vi "Dashboard Main.vi"() -> ()   [LabVIEW 2014]
uses:
  <vilib>/event_ctls.llb/eventvkey.ctl
  <vilib>/Rock Robotics/WPI/Dashboard/WPI_DashboardLogging Global.vi
  <vilib>/Rock Robotics/Network Tables/SD Write Number.vi
  <vilib>/Rock Robotics/Network Tables/SD Read Number.vi
  <vilib>/Utility/config.llb/Write Key (String).vi
  <vilib>/Utility/config.llb/Write Key (I32).vi
  <vilib>/Utility/config.llb/NI_LVConfig.lvlib
panel:
  out "Numeric Array":dbl[](array[numeric])
  in  "TCP":refnum<k5>
  in  "Rec Mode":enum32{"Stop", "Record", "Playback"}(radio)
  in  "Vision":u16(ring) items=["Camera Off", "USB Camera SW", "USB Camera HW", "IP Camera"]
  out "Camera IP":string
  out "Image Message":string="Timeout in Camera Communications"
  in  "Dashboard Tab":T1(tab)
  out "pot":dbl(slide) scale=0.0..30.0
  in  "LED_Off":u32(colorbox)=65282
  in  "Camera Settings":T2={"Frame Rate"=30, "Compression"=30, "Size"=1} {"Frame Rate" scale=1.0..30.0; "Size" items=["640x480", "320x240", "160x120"]}
  out "MotorChart R":cluster{"Numeric":dbl, "Numeric":dbl}(graph)
  out "MotorChart L":T3(graph)
  out "MotorSliders R":cluster{"MotorSlide1":dbl, "MotorSlide2":dbl} {"MotorSlide2" scale=-1.0..1.0 scale format="%#_2e"; "MotorSlide1" scale=-1.0..1.0 scale format="%#_2e"}
  out "MotorSliders L":T4 {"MotorSlide4 2" scale=0.0..14.0 scale format="%#_2e"; "MotorSlide2" scale=-1.0..1.0 scale format="%#_2e"; "MotorSlide1" scale=-1.0..1.0 scale format="%#_2e"}
  out "Gyro":dbl(knob) scale=0.0..360.0
  out "JS1 Z":dbl(slide) scale=-1.0..1.0 scale format="%#_2e"
  out "JS1 Graph":cluster{"X":dbl, "Y":dbl}[](graph)
  out "JS1 Buttons":T5
  out "JS2 Z":dbl(slide) scale=-1.0..1.0 scale format="%#_2e"
  out "JS2 Graph":cluster{"X":dbl, "Y":dbl}[](graph)
  out "JS2 Buttons":T5
  out "Mode":T6(ring)=enum."Auto Disabled"
  in  "DB Camera Config":bool
  out "fps":dbl format="%#.1g"
  out "Mbps":dbl format="%#.1g"
  out "Mbps 2":bool
  in  "LED_On":u32(colorbox)=1535
  in  "DB/String 9":string
  in  "DB/String 8":string
  in  "DB/String 7":string
  in  "DB/String 6":string
  in  "DB/String 5":string
  in  "DB/String 4":string
  in  "DB/String 3":string
  in  "DB/String 2":string
  in  "DB/String 1":string
  in  "DB/String 0":string
  in  "DB/Slider 0":dbl(slide) scale=0.0..5.0
  in  "DB/Slider 1":dbl(slide) scale=0.0..5.0
  in  "DB/Slider 2":dbl(slide) scale=0.0..5.0
  in  "DB/Slider 3":dbl(slide) scale=0.0..5.0
  out "DB/LED 3":bool
  out "DB/LED 2":bool
  out "DB/LED 1":bool
  out "DB/LED 0":bool
  in  "DB/Button 3":bool
  in  "DB/Button 2":bool
  in  "DB/Button 1":bool
  in  "DB/Button 0":bool caption="New Name"
  in  "Test Slider":dbl(slide) scale=0.0..100.0 scale format="%#_3g"
  in  "On/Off":bool caption="Solenoid"
  in  "Test Name":u16(ring) items=["Select the test to run...", "Example Test", "-------------------------------", "List of tests is built in robot code.", "Replace with your own automated tests."]
  in  "Test Tree":string(tree)
  in  "Motor":cluster{"Value":dbl, "Enable":bool} {"Value" scale=-1.0..1.0 scale format="%#_3g"}
  out "Progress":T7 {"Test Progress" scale=0.0..100.0}
  in  "Rev/Fwd":cluster{"Forward":bool, "Reverse":bool}
  in  "Test Ring":u16(ring) items=["Monochrome", "Color"]
  in  "Listbox":i32(listbox)
  out "Tree":string(tree)
  out "Camera Image":T8(plugin-control)
  out "Boolean":bool
  # "Left"
  # "Front"
  # "Right"
  # "Battery"
  # "This tab is a great place for autonomous settings and robot-specific values.\nPlace controls and indicators inside this tab and match name to\nDashboard Variables on robot. You can also delete this comment."
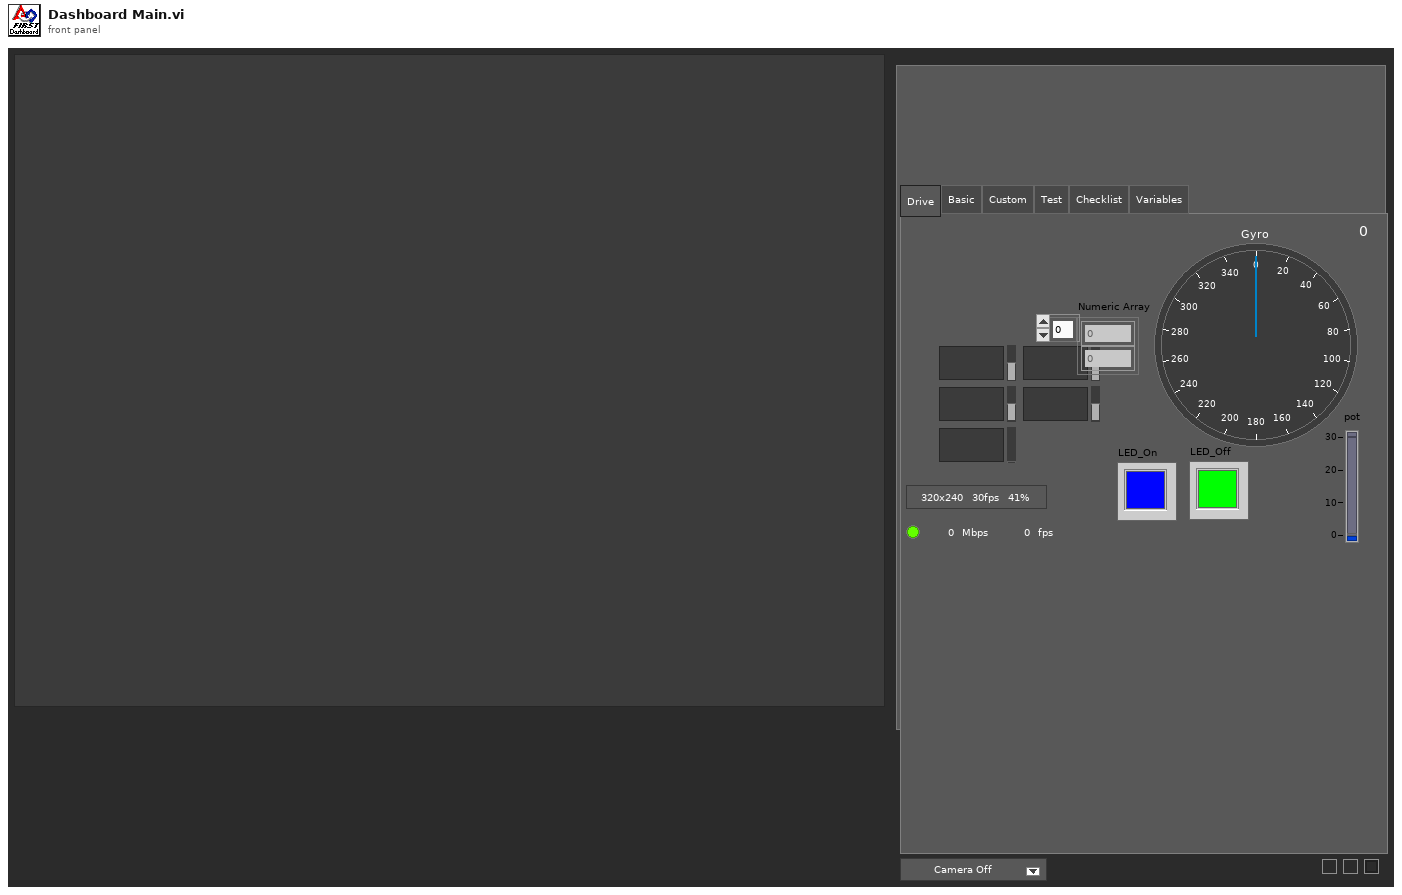
[diagram p1: front panel]
types:
  T1 = enum32{"Drive", "Basic", "Custom", "Test", "Checklist", "Variables"}
  T2 = cluster{"Frame Rate":i32, "Compression":i32, "Size":u16}
  T3 = cluster{"Numeric":dbl, "Numeric":dbl, "Battery V":dbl}
  T4 = cluster{"MotorSlide1":dbl, "MotorSlide2":dbl, "MotorSlide4 2":dbl}
  T5 = cluster{bool, bool, bool, bool, bool, bool, bool, bool, bool, bool, bool, bool}
  T6 = enum8{"Tele-Op Disabled", "Tele-Op Enabled", "Auto Disabled", "Auto Enabled", "Test Disabled", "Test Enabled", "Disconnected", "No Code", "E-Stop"}
  T7 = cluster{"Test Progress":u8, "Test Progress Text":string}
  T8 = typedef "IMAQ Image.ctl" = refnum<image>
  T9 = typedef "Image Type" = u32
  T10 = cluster{"Camera Image":refnum<vi>, "Dashboard Tab":refnum<vi>, "Boolean":refnum<vi>, "Vision":refnum<vi>, "Rec Mode":refnum<vi>, "Test Slider":refnum<vi>, "On/Off ":refnum<vi>, "Test Ring":refnum<vi>, "Rev/Fwd":refnum<vi>, "Test Name":refnum<vi>, "Motor":refnum<vi>, "Progress":refnum<vi>, "CheckList":refnum<vi>, "Tree":refnum<vi>, "Test Tree":refnum<vi>}
  T11 = cluster{"Error Strings":string, "Disable Counts":cluster{u16, u16}, "Rail Faults":cluster{u16, u16, u16}, "Robot IP":string, "DB Mode":u8, "Event Info":cluster{"Name":string, "Type":u8, "Number":u16, "Replay":u8}, "Camera Addr":string}
  T12 = cluster{"Storage":cluster{"Disk Free":u64, "RAM Block":u32, "RAM free":u32}, "CPU Utilization":cluster{"CPU % ISR":sgl, "CPU % Time Crit":sgl, "CPU % Timed Str":sgl, "CPU % High":sgl, "CPU % Above":sgl, "CPU % Normal":sgl, "CPU % Low":sgl}, "CAN":cluster{"% Bus Utilization":sgl, "Bus Off Cnt":u32, "TX_FIFO Full Cnt":u32, "Receive Error Cnt":u8, "Transmit Error Cnt":u8}, "HID":cluster{"HID Outputs":u32, "Rumble Low":u16, "Rumble High":u16}[]}
  T13 = cluster{"Status bits":cluster{"Test Mode":bool, "Autonomous":bool, "Enabled":bool, "Code Start":bool, "Brownout":bool, "Reserved 2":bool, "Reserved 3":bool, "E-Stop":bool}, "Code Trace":cluster{"Disabled":bool, "TeleOp":bool, "Auto":bool, "Test":bool}, "Controller Type":enum16{"unknown", "cRIO", "roboRio"}, "Code?":enum16{"unknown", "noCode", "code"}, "Battery V":dbl}
  T14 = cluster{"Control Bits":cluster{"TestMode":bool, "Autonomous":bool, "Enabled":bool, "FMS Present":bool, bool, bool, bool, "E-Stop":bool}, "Team Station ":u8, "Countdown":sgl, "Joystick Values":cluster{"Axes":dbl[], "Buttons":bool[], "POVs":i16[]}[]}
  T15 = cluster{"Axes":dbl[], "Buttons":bool[], "POVs":i16[]}[]
  T16 = cluster{"Axes":dbl[], "Buttons":bool[], "POVs":i16[]}
  T17 = cluster{"Buttons[0]":bool, "Buttons[1]":bool, "Buttons[2]":bool, "Buttons[3]":bool, "Buttons[4]":bool, "Buttons[5]":bool, "Buttons[6]":bool, "Buttons[7]":bool, "Buttons[8]":bool, "Buttons[9]":bool, "Buttons[10]":bool, "Buttons[11]":bool}
  T18 = typedef "NI_LVConfig.lvlib/Config Data RefNum.ctl" = refnum<k1>
  T19 = cluster{"Operation":enum16{"Update", "Clear"}, "Color Box":u32}[]
  T20 = typedef "eventvkey.ctl" = enum16{"ASCII", "Enter", "Return", "Shift", "Ctrl", "Alt", "Cmd", "Opt", "Caps", "NumLock", "Clear", "Break", "Up", "Down", "Left", "Right", "Insert", "Delete", "Home", "End", "PageUp", "PageDown", "Escape", "Help", "Pause", "ScrollLock", "F1", "F2", "F3", "F4", "F5", "F6", "F7", "F8", "F9", "F10", "F11", "F12", "F13", "F14", "F15", "F16", "F17", "F18", "F19", "F20", "F21", "F22", "F23", "F24", "Play", "VolumeUp", "VolumeDown", "Mute", "Two Byte Char"}
  T21 = cluster{"Image Size":bool, "Image Type":bool, "Pixel Value":bool, "ROI Information":bool, "Zoom Factor":bool}
  T22 = enum8{"Enabled", "Disabled", "Disabled and Grayed Out"}
  T23 = cluster{"Operation":enum16{"Update", "Clear"}, "Color Box":u32}
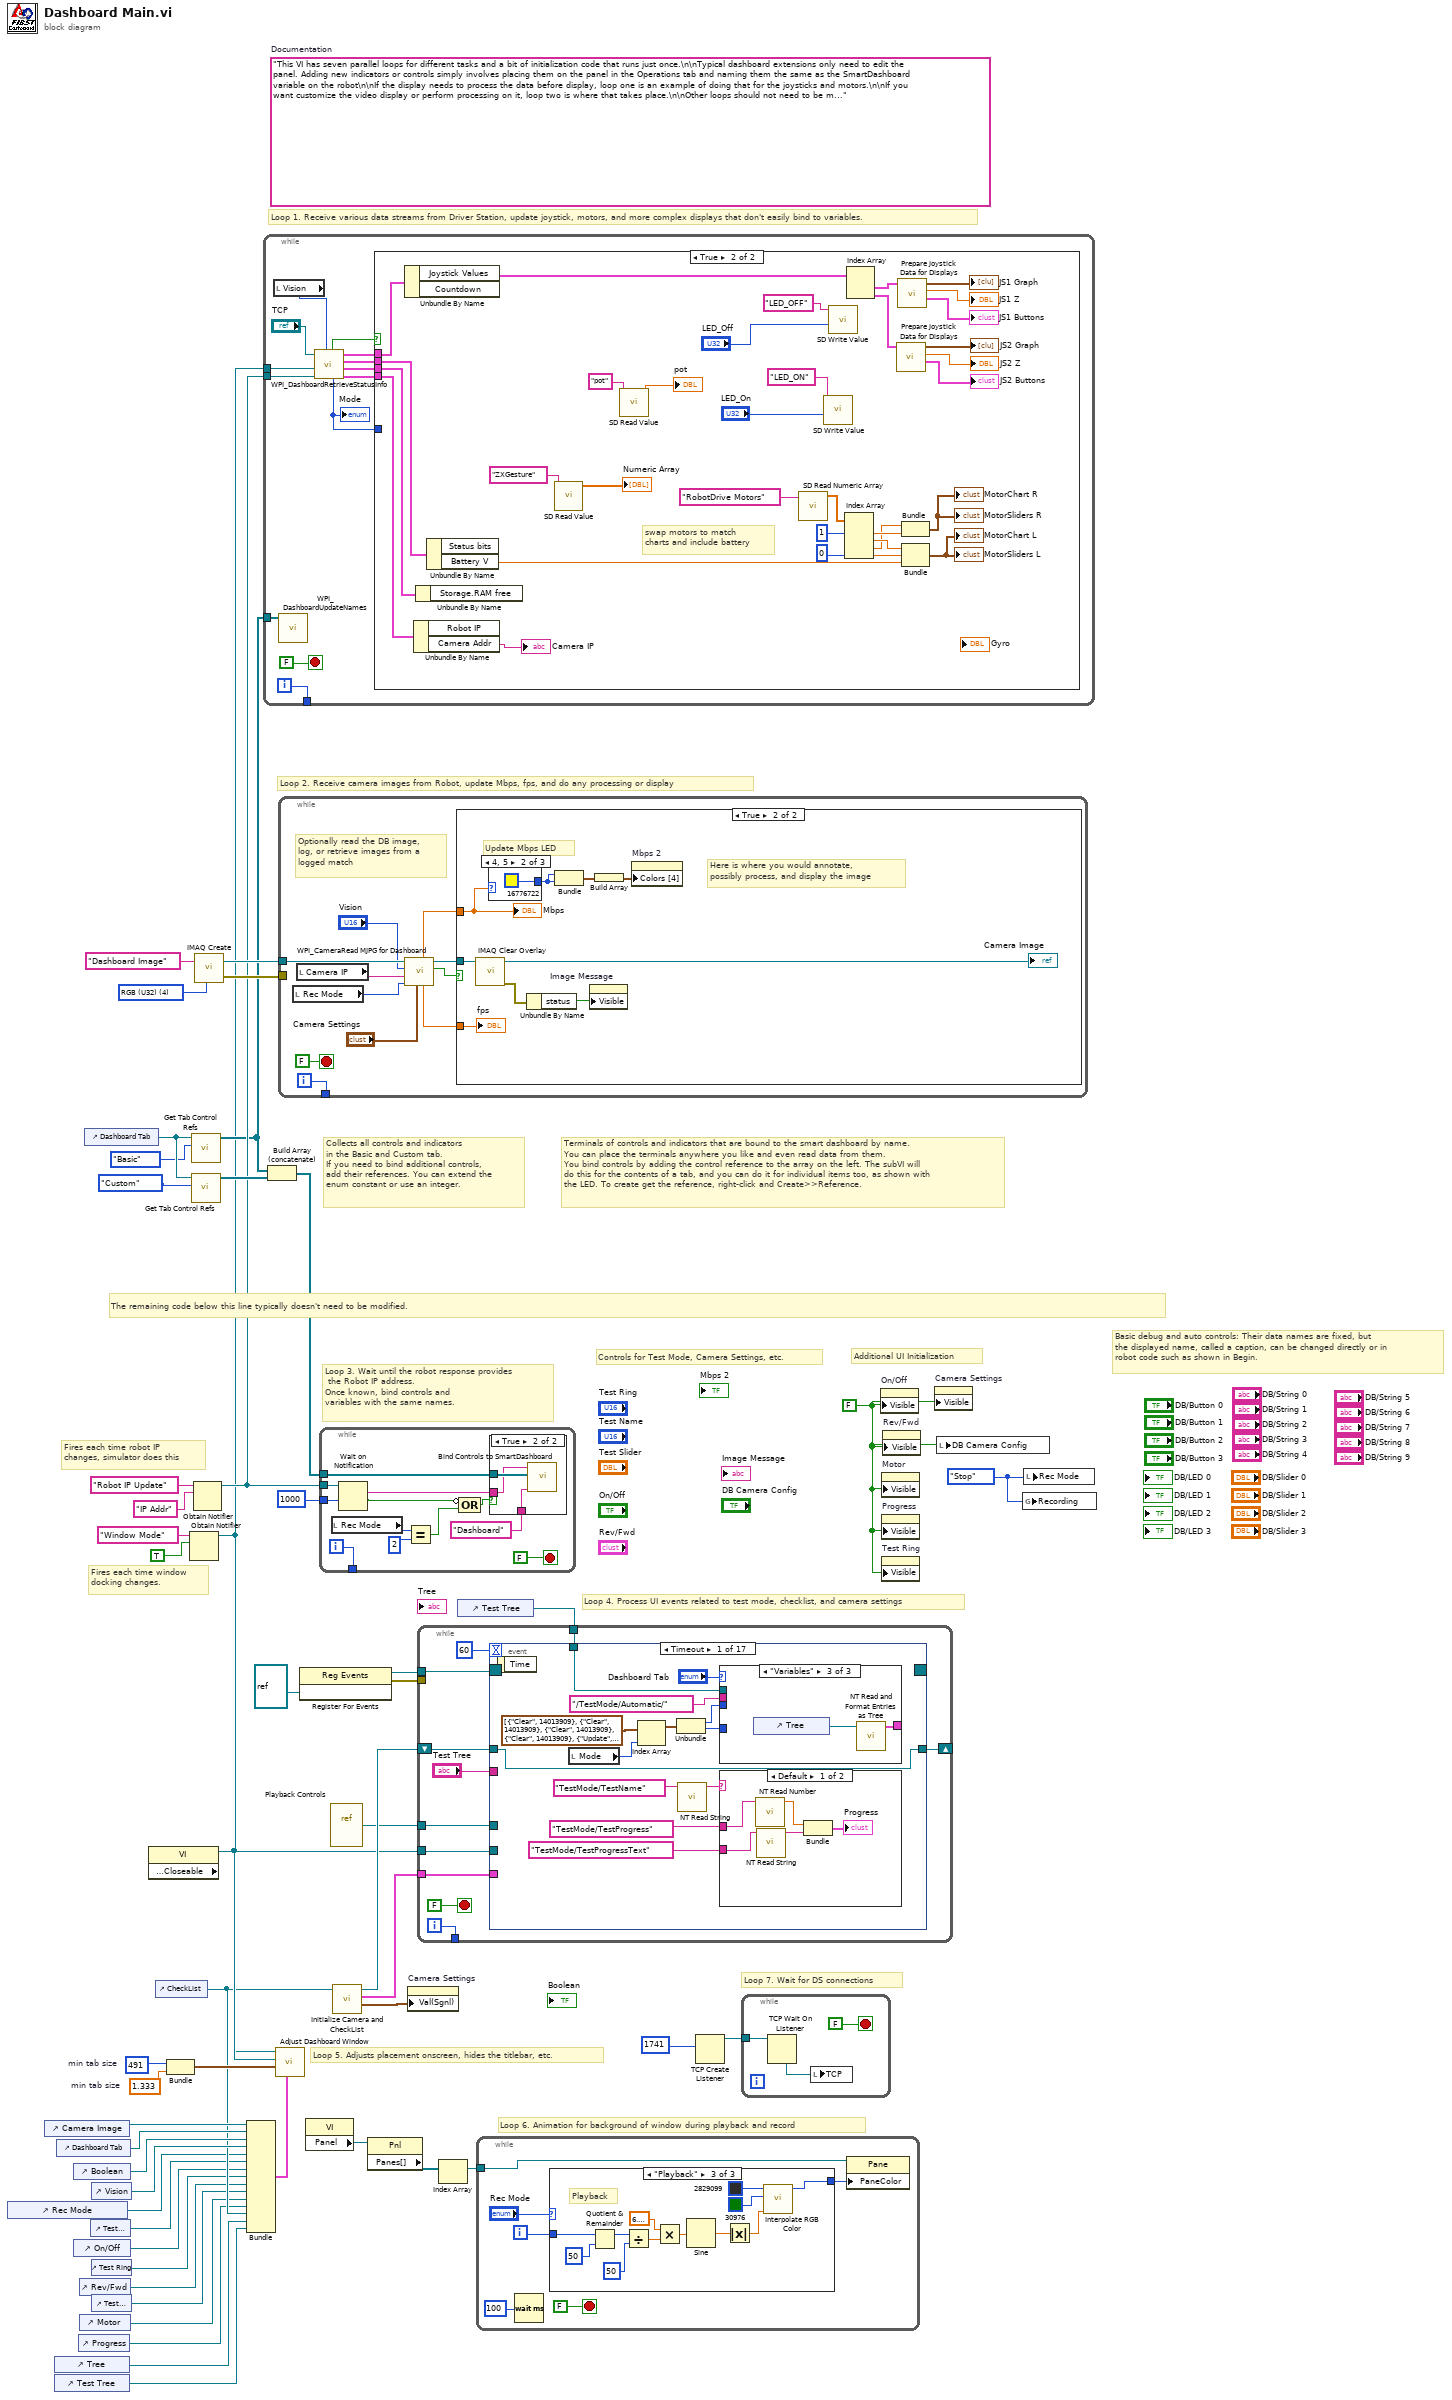
[diagram p0: block diagram]
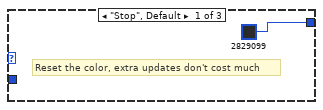
[diagram p3: hidden frame]
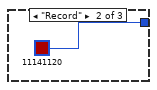
[diagram p4: hidden frame]
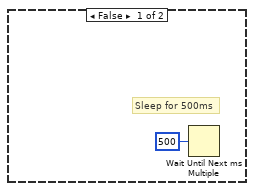
[diagram p6: hidden frame]
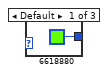
[diagram p7: hidden frame]
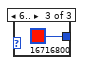
[diagram p8: hidden frame]
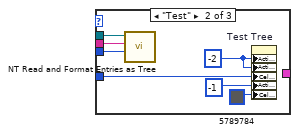
[diagram p10: hidden frame]
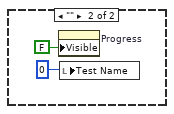
[diagram p11: hidden frame]
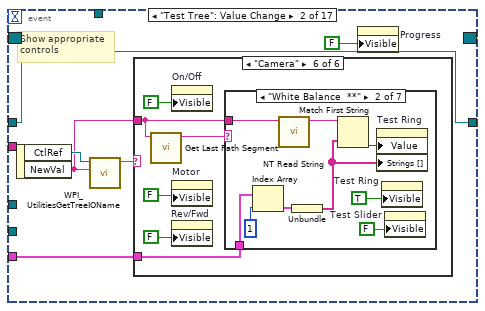
[diagram p12: hidden frame]
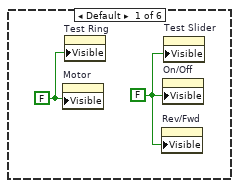
[diagram p13: hidden frame]
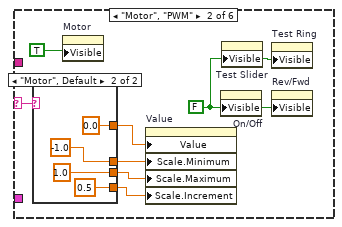
[diagram p14: hidden frame]
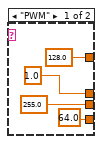
[diagram p15: hidden frame]
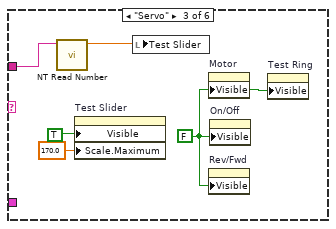
[diagram p16: hidden frame]
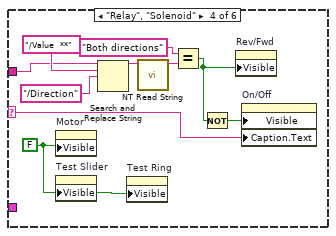
[diagram p17: hidden frame]
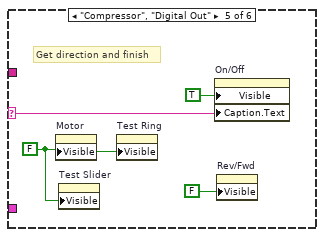
[diagram p18: hidden frame]
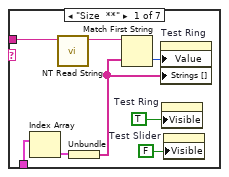
[diagram p19: hidden frame]
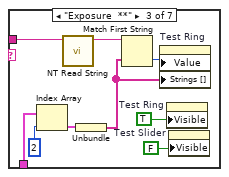
[diagram p20: hidden frame]
diagram:
  w24 = 491  # min tab size
  w23 = 1.333  # min tab size
  w32 = enum32{"Stop", "Record", "Playback"}."Stop" ("Rec Mode")
  w6 = FALSE ("Visible")
  (unwired) "This VI has seven parallel loops for different tasks and a bit of initialization code that runs just once.\n\nTypical dashboard extensions only need to edit the panel. Adding new indicators or controls simply involves placing them on the panel in the Operations tab and naming them the same as the SmartDashboard variable on the robot\n\nIf the display needs to process the data before display, loop one is an example of doing that for the joysticks and motors.\n\nIf you want customize the video display or perform processing on it, loop two is where that takes place.\n\nOther loops should not need to be modified. They are pretty standard, and document the task they perform."  # Documentation
  w52 = T9 4 items=["Grayscale (U8)", "Grayscale (I16)", "Grayscale (SGL)", "Complex (CSG)", "RGB (U32)", "HSL (U32)", "RGB (U64)"] ("Image Type")
  # "Loop 7. Wait for DS connections"
  # "Basic debug and auto controls: Their data names are fixed, but\nthe displayed name, called a caption, can be changed directly or in\nrobot code such as shown in Begin."
  # "Controls for Test Mode, Camera Settings, etc."
  # "Additional UI Initialization"
  # "Loop 6. Animation for background of window during playback and record"
  # "Fires each time robot IP\nchanges, simulator does this"
  # "Fires each time window\ndocking changes."
  # "Collects all controls and indicators\nin the Basic and Custom tab.\nIf you need to bind additional controls,\nadd their references. You can extend the\nenum constant or use an integer."
  # "The remaining code below this line typically doesn't need to be modified."
  # "Loop 4. Process UI events related to test mode, checklist, and camera settings"
  # "Terminals of controls and indicators that are bound to the smart dashboard by name.\nYou can place the terminals anywhere you like and even read data from them.\nYou bind controls by adding the control reference to the array on the left. The subVI will\ndo this for the contents of a tab, and you can do it for individual items too, as shown with\nthe LED. To create get the reference, right-click and Create>>Reference."
  # "Loop 3. Wait until the robot response provides\n the Robot IP address.\nOnce known, bind controls and\nvariables with the same names."
  # "Loop 5. Adjusts placement onscreen, hides the titlebar, etc."
  # "Loop 1. Receive various data streams from Driver Station, update joystick, motors, and more complex displays that don't easily bind to variables."
  # "Loop 2. Receive camera images from Robot, update Mbps, fps, and do any processing or display"
  n1 = control-ref of="Rec Mode"() -> (w12:refnum<vi>)
  n2 = control-ref of="Camera Image"() -> (w27:refnum<vi>)
  n3 = control-ref of="Tree"() -> (w16:refnum<vi>)
  n4 = control-ref of="Test Tree"() -> (w15:refnum<vi>)
  n5 = control-ref of="Dashboard Tab"() -> (w26:refnum<vi>)
  n6 = control-ref of="Boolean"() -> (w21:refnum<vi>)
  n7 = control-ref of="On/Off"() -> (w10:refnum<vi>)
  n8 = control-ref of="Progress"() -> (w7:refnum<vi>)
  n9 = control-ref of="Rev/Fwd"() -> (w8:refnum<vi>)
  n10 = control-ref of="Motor"() -> (w13:refnum<vi>)
  n11 = control-ref of="Dashboard Tab"() -> (w30:refnum<vi>)
  n12 = control-ref of="Test Slider"() -> (w11:refnum<vi>)
  n13 = control-ref of="Vision"() -> (w25:refnum<vi>)
  n14 = control-ref of="Test Ring"() -> (w9:refnum<vi>)
  n15 = control-ref of="Test Name"() -> (w14:refnum<vi>)
  n16 = property class="VI" props=["Front Panel.Closeable"]() -> (reference out=w31:refnum<vi>)  [unwired: 2 in, 2 out]
  n17 = control-ref of="CheckList"() -> (w17:refnum<vi>)
  n18 = Bundle("min tab size"=w24, "min tab size"=w23) -> (w22:cluster{"min tab size":i32, "min tab size":dbl})  [unwired: 1 in]
  n19 = Obtain Notifier(name (unnamed)="Window Mode", notification data type=TRUE) -> (notifier out=w3:refnum<notifier>)  [unwired: 2 in, 2 out]
  n20 = call <vilib>:"Get Tab Control Refs.vi"("Page Index"=T1."Basic" ("Dashboard Tab"), "TabControl in"=w30) -> ("ControlsOnPage"=w4:refnum<vi>[])  [unwired: 9 in]
  n21 = call <vilib>:"Get Tab Control Refs.vi"("Page Index"=T1."Custom" ("Dashboard Tab"), "TabControl in"=w30) -> ("ControlsOnPage"=w29:refnum<vi>[])  [unwired: 9 in]
  n22 = Obtain Notifier(name (unnamed)="Robot IP Update", notification data type="IP Addr" ("name (unnamed)")) -> (notifier out=w5:refnum<notifier>)  [unwired: 2 in, 2 out]
  n23 = call "IMAQ Create"("Image Name"="Dashboard Image", "Image Type"=w52) -> ("New Image"=w50:T8, "error out"=w49:errorcluster)  [unwired: 2 in, 1 out]
  n24 = Bundle("Camera Image"=w27, "Dashboard Tab"=w26, "Boolean"=w21, "Vision"=w25, "Rec Mode"=w12, "Test Slider"=w11, "On/Off"=w10, "Test Ring"=w9, "Rev/Fwd"=w8, "Test Name"=w14, "Motor"=w13, "Progress"=w7, "CheckList"=w17, "Tree"=w16, "Test Tree"=w15) -> (w18:T10)  [unwired: 1 in]
  n25 = while {
    tunnel: [w64] -> _
    tunnel: w5 -> [w58]
    tunnel: w4 -> [w57]
    tunnel: w3 -> [w53]
    i -> [w64]
    stop <- FALSE stop-if-true
    n26 = local read "Vision"() -> (w55:u16)
    n27 = call <vilib>:"WPI_DashboardUpdateNames.vi"("Controls on Tab"=w57) -> ()  [unwired: 11 in]
    n28 = call <vilib>:"WPI_DashboardRetrieveStatusInfo.vi"("Vision"=w55, "Binding Refnum"=w58, "Window Mode Notifier"=w53, "TCP Cnx"="TCP") -> ("Power and Errors"=w59:T11, "Robot Metrics"=w62:T12, "Status Info"=w63:T13, "Control Info"=w60:T14, "Robot Mode"=w56:T6, "Process?"=w61:bool)  [unwired: 2 in]
    "Mode" <- w56
    n29 = case shown="True" w61 {
      tunnel: w63 -> [_ w98]
      tunnel: w62 -> [_ w97]
      tunnel: w60 -> [_ w96]
      tunnel: w59 -> [_ w95]
      tunnel: w56 -> [_ _]
      frame False {
      }
      frame True {
        # "swap motors to match\ncharts and include battery"
        n30 = Unbundle By Name(w96) -> ("Joystick Values"=w83:T15)  [unwired: 1 out]
        n31 = Unbundle By Name(w95) -> ("Camera Addr"=→"Camera IP":string)  [unwired: 1 out]
        n32 = Unbundle By Name(w97) -> ()  [unwired: 1 out]
        n33 = Unbundle By Name(w98) -> ("Battery V"=w84:dbl)  [unwired: 1 out]
        n34 = call-poly <vilib>:"SD Read Value.vi"("Name"="ZXGesture") -> ("Numeric Array"=→"Numeric Array":dbl[])  [unwired: 8 in, 2 out]
        n35 = call-poly <vilib>:"SD Read Value.vi"("Name"="pot") -> ("Numeric"=→"pot":dbl)  [unwired: 8 in, 2 out]
        n36 = call <vilib>:"SD Read Numeric Array.vi"("Name"="RobotDrive Motors") -> ("Numeric Array"=w86:dbl[])  [unwired: 8 in, 2 out]
        n37 = call-poly <vilib>:"SD Write Value.vi"("Numeric"="LED_On", "Name"="LED_ON") -> ()  [unwired: 8 in, 2 out]
        n38 = call-poly <vilib>:"SD Write Value.vi"("Numeric"="LED_Off", "Name"="LED_OFF") -> ()  [unwired: 8 in, 2 out]
        n39 = Index Array(array=w86, index #1=1, index #4=0) -> (element #1=w90:dbl, element #2=w91:dbl, element #3=w89:dbl, element #4=w94:dbl)  [unwired: 2 in]
        n40 = Index Array(array=w83) -> (element #1=w82:T16, element #2=w77:T16)  [unwired: 2 in]
        n41 = call "Prepare Joystick Data for Displays.vi"("Joystick Values"=w77) -> ("Buttons"=→"JS2 Buttons":T17, "Z Axis"=→"JS2 Z":dbl, "Cartesian Data"=→"JS2 Graph":cluster{"X axis":dbl, "X axis":dbl}[])  [unwired: 8 in]
        n42 = call "Prepare Joystick Data for Displays.vi"("Joystick Values"=w82) -> ("Buttons"=→"JS1 Buttons":T17, "Z Axis"=→"JS1 Z":dbl, "Cartesian Data"=→"JS1 Graph":cluster{"X axis":dbl, "X axis":dbl}[])  [unwired: 8 in]
        n43 = Bundle("Numeric"=w89, "Numeric"=w90) -> (→"MotorChart R" →"MotorSliders R":cluster{"Numeric":dbl, "Numeric":dbl})  [unwired: 1 in]
        n44 = Bundle("Numeric"=w91, "Numeric"=w94, "Battery V"=w84) -> (→"MotorChart L" →"MotorSliders L":T3)  [unwired: 1 in]
      }
    }
  }
  n45 = Build Array (concatenate)(w4, w29) -> (w28:refnum<vi>[])
  n46 = call "Adjust Dashboard Window.vi"("Sizing Refnums"=w18, "Size Constraints"=w22, "VI"=w31, "Notifier in"=w3) -> ()  [unwired: 8 in]
  n47 = while {
    tunnel: w50 -> [w107]
    tunnel: w49 -> [_]
    tunnel: [w108] -> _
    i -> [w108]
    stop <- FALSE stop-if-true
    # "Optionally read the DB image,\nlog, or retrieve images from a\nlogged match"
    n48 = local read "Rec Mode"() -> (w101:enum32{"Stop", "Record", "Playback"})
    n49 = local read "Camera IP"() -> (w99:string)
    n50 = call <vilib>:"WPI_CameraRead MJPG for Dashboard.vi"("Camera Settings"="Camera Settings", "Rec Mode"=w101, "Camera IP"=w99, "Camera Mode"="Vision", "Refnum in"=w107) -> ("Active"=w105:bool, "Refnum out"=w106:T8, "FPS"=w104:dbl, "Bandwidth (Mbps)"=w103:dbl)  [unwired: 3 in]
    n51 = case shown="True" w105 {
      tunnel: w106 -> [_ w114]
      tunnel: w103 -> [_ w113]
      tunnel: w104 -> [_ w111]
      frame False {
        # "Sleep for 500ms"
        n52 = Wait Until Next ms Multiple(millisecond multiple=u32 500) -> ()  [unwired: 1 out]
      }
      frame True {
        # "Here is where you would annotate,\npossibly process, and display the image"
        # "Update Mbps LED"
        n53 = call "IMAQ Clear Overlay"("Image"=w114) -> ("error out"=w118:errorcluster, "Image Out"=→"Camera Image":T8)  [unwired: 2 in, 7 out]
        n54 = case shown="4, 5" w113 {
          tunnel: [u32 6618880 ("Color Box") u32 16776722 ("Color Box") u32 16716800 ("Color Box")] -> w115
          frame Default {
          }
          frame 4, 5 {
          }
          frame 6.. {
          }
        }
        n55 = Unbundle By Name(w118) -> ("status"=w119:bool)
        n56 = Bundle("Color Box"=w115, "Color Box"=w115) -> (w117:cluster{"Color Box":u32, "Color Box":u32})  [unwired: 1 out]
        n57 = property on="Image Message" class="Str"("Visible"=w119) -> ()  [unwired: 2 in, 2 out]
        n58 = Build Array(w117) -> (w116:cluster{"Color Box":u32, "Color Box":u32}[])
        n59 = property on="Mbps 2" class="Bool (strict)"("Colors [4]"=w116) -> ()  [unwired: 2 in, 2 out]
        "Mbps" <- w113
        "fps" <- w111
      }
    }
  }
  n60 = register-events(refnum<vi> refnum) -> (reference out=w36:refnum<event-registration>, error out=w35:errorcluster)  [unwired: 2 in]
  n61 = property class="VI"() -> ("Panel"=w39:refnum<vi>)  [unwired: 2 in, 2 out]
  n62 = while {
    tunnel: w28 -> [w134]
    tunnel: w5 -> [w132]
    tunnel: [w130] -> _
    tunnel: u32 1000 ("milliseconds to wait") -> [w129]
    i -> [w130]
    stop <- FALSE stop-if-true
    n63 = local read "Rec Mode"() -> (w125:enum32{"Stop", "Record", "Playback"})
    n64 = Wait on Notification(notifier=w132, timeout in ms (-1)=w129) -> (notification=w131:string, timed out?=w127:bool)  [unwired: 2 in, 2 out]
    n65 = Equal?(x=w125, y=u16 2 ("Rec Mode")) -> (x = y?=w126:bool)
    n66 = Compound Arithmetic op=OR(invert w127, w126) -> (w128:bool)
    n67 = case shown="True" w128 {
      tunnel: w134 -> [_ w137]
      tunnel: w131 -> [_ w136]
      tunnel: "Dashboard" -> [_ w135]
      frame False {
      }
      frame True {
        n68 = call <vilib>:"Bind Controls to SmartDashboard.vi"("Client Name"=w135, "Bound Control Refs"=w137, "Server IP Address"=w136) -> ()  [unwired: 9 in]
      }
    }
  }
  n69 = vi-ref "Playback Controls.vi"() -> (w37:refnum<vi>)
  n70 = call "Initialize Camera and CheckList.vi"("ListBox in"=w17) -> ("Cluster"=w43:cluster{"value":i32, "value":i32, "index":i32}, "Array"=w44:cluster{string[]}[], "File Refnum"=w42:T18)  [unwired: 8 in]
  n71 = property class="Pnl"(reference=w39) -> ("Panes[]"=w40:refnum<vi>[])  [unwired: 1 in, 2 out]
  n72 = property on="Camera Settings" class="Clust (strict)"("Val(Sgnl)"=w43) -> ()  [unwired: 2 in, 2 out]
  n73 = Index Array(array=w40) -> (element=w38:refnum<vi>)  [unwired: 1 in]
  n74 = control-ref of="Test Tree"() -> (w41:refnum<vi>)
  n75 = while {
    tunnel: w44 -> [w145]
    shift-right: [w144] -> _
    shift-left: w42 -> [w143]
    tunnel: [w142] -> _
    tunnel: w41 -> [w141]
    tunnel: w37 -> [w140]
    tunnel: w36 -> [w139]
    tunnel: w35 -> [_]
    tunnel: w31 -> [w138]
    i -> [w142]
    stop <- FALSE stop-if-true
    n76 = event shown="[0] Timeout" {
      selector: w139 -> [_ _ _ _ _ _ _ _ _ _ _ _ _ _ _ _ _]
      dyn-events: [_ _ _ _ _ _ _ _ _ _ _ _ _ w383 _ _ _] -> _
      timeout: u32 60 ("milliseconds to wait") -> [_ _ _ _ _ _ _ _ _ _ _ _ _ _ _ _ _]
      tunnel: w141 -> [w157 _ _ _ _ _ _ _ _ _ _ _ _ _ _ _ _]
      tunnel: "Test Tree" -> [_ _ _ _ _ _ _ _ w352 w360 w362 w366 w374 _ _ _ _]
      tunnel: w145 -> [_ w179 _ _ _ _ w316 w346 _ _ _ _ _ _ _ _ _]
      tunnel: [w153 w178 w277 w282 w290 w302 w315 w339 w351 w358 w361 w365 w373 w385 w399 w400 w410] -> w144
      tunnel: w143 -> [w153 w178 w277 w282 w290 w302 w314 w339 w351 w358 w361 w365 w373 w385 w399 w400 w410]
      tunnel: w140 -> [_ _ _ _ _ _ _ _ _ _ _ _ _ w386 _ w403 _]
      tunnel: w138 -> [_ _ _ _ _ _ _ _ _ _ _ _ _ w381 _ _ _]
      event Timeout {
        n77 = event-data() -> ()  [unwired: 1 in, 1 out]
        n78 = local read "Mode"() -> (w156:T6)
        n79 = Index Array(array=T19 [{"Operation"=enum."Clear", "Color Box"=14013909}, {"Operation"=enum."Clear", "Color Box"=14013909}, {"Operation"=enum."Clear", "Color Box"=14013909}, {"Operation"=enum."Clear", "Color Box"=14013909}, {"Operation"=enum."Update", "Color Box"=14013909}, {"Operation"=enum."Update", "Color Box"=16777215}, {"Operation"=enum."Clear", "Color Box"=14013909}, {"Operation"=enum."Clear", "Color Box"=14013909}, {"Operation"=enum."Clear", "Color Box"=14013909}], index=w156) -> (element=w151:T23)
        n80 = Unbundle(w151) -> ("Operation"=w150:enum16{"Update", "Clear"}, "Color Box"=w149:u32)
        n81 = call <vilib>:"NT Read String.vi"("Name"="TestMode/TestName") -> ("String"=w160:string)  [unwired: 9 in, 1 out]
        n82 = case shown="\"Variables\"" "Dashboard Tab" {
          tunnel: w157 -> [_ w168 _]
          tunnel: "/TestMode/Automatic/" ("Name Pattern") -> [_ w167 _]
          tunnel: w150 -> [_ w166 _]
          tunnel: [_ _ w170] -> _
          tunnel: w149 -> [_ w162 _]
          frame "Custom", Default {
          }
          frame "Test" {
            w165 = -2 ("Active Item:Row Number")
            n83 = call <vilib>:"NT Read and Format Entries as Tree.vi"("Operation"=w166, "Name Pattern"=w167, "Tree Refnum"=w168) -> ()  [unwired: 7 in, 2 out]
            n84 = property on="Test Tree" class="Tree (strict)"("Active Item Row Number"=w165, "ActiveColNum"=w165, "CellBG"=w162, "Active Item Row Number"=-1 ("Active Item:Row Number"), "CellBG"=u32 5789784 ("Color Box")) -> ()  [unwired: 2 in, 2 out]
          }
          frame "Variables" {
            n85 = control-ref of="Tree"() -> (w169:refnum<vi>)
            n86 = call <vilib>:"NT Read and Format Entries as Tree.vi"("Tree Refnum"=w169) -> ("Formatted Strings"=w170:cluster{"Name":string, "Value":string}[])  [unwired: 9 in, 1 out]
          }
        }
        n87 = case shown="Default" w160 {
          tunnel: "TestMode/TestProgress" ("Name") -> [w172 _]
          tunnel: "TestMode/TestProgressText" ("Name") -> [w171 _]
          frame Default {
            n88 = call <vilib>:"NT Read Number.vi"("Name"=w172) -> ("Numeric"=w173:dbl)  [unwired: 9 in, 1 out]
            n89 = call <vilib>:"NT Read String.vi"("Name"=w171) -> ("String"=w174:string)  [unwired: 9 in, 1 out]
            n90 = Bundle("Numeric"=w173, "String"=w174) -> (→"Progress":cluster{"Numeric":dbl, "String":string})  [unwired: 1 in]
          }
          frame "" {
            n91 = property on="Progress" class="Clust (strict)"("Visible"=FALSE) -> ()  [unwired: 2 in, 2 out]
            n92 = local write "Test Name"(u16 0) -> ()
          }
        }
      }
      event "Test Tree": Value Change {
        # "Show appropriate\ncontrols"
        n93 = event-data() -> ("CtlRef"=w182:refnum<vi>, "NewVal"=w180:string)  [unwired: 1 in]
        n94 = call <vilib>:"WPI_UtilitiesGetTreeIOName.vi"("NewVal"=w180, "TreeControl in"=w182) -> ("I/O Name"=w183:string)  [unwired: 9 in]
        n95 = case shown="\"Camera\"" w183 {
          selector: w183 -> [_ w190 _ w208 w217 _]
          tunnel: w180 -> [_ _ w205 w207 _ w224]
          tunnel: w179 -> [_ _ _ _ _ w223]
          frame Default {
            w185 = FALSE ("Visible")
            w184 = FALSE ("Visible")
            n96 = property on="Motor" class="Clust (strict)"("Visible"=w184) -> ()  [unwired: 2 in, 2 out]
            n97 = property on="Test Ring" class="Ring (strict)"("Visible"=w184) -> ()  [unwired: 2 in, 2 out]
            n98 = property on="Rev/Fwd" class="Clust (strict)"("Visible"=w185) -> ()  [unwired: 2 in, 2 out]
            n99 = property on="On/Off" class="Bool (strict)"("Visible"=w185) -> ()  [unwired: 2 in, 2 out]
            n100 = property on="Test Slider" class="Slide (strict)"("Visible"=w185) -> ()  [unwired: 2 in, 2 out]
          }
          frame "Motor", "PWM" {
            w191 = FALSE ("Visible")
            n101 = case shown="\"Motor\", Default" w190 {
              tunnel: [1.0 ("Value") -1.0 ("Value")] -> w189
              tunnel: [255.0 ("Value") 1.0 ("Value")] -> w188
              tunnel: [128.0 ("Value") 0.0 ("Value")] -> w187
              tunnel: [64.0 ("Value") 0.5 ("Value")] -> w186
              frame "PWM" {
              }
              frame "Motor", Default {
              }
            }
            n102 = property on="Motor" class="Clust (strict)"("Visible"=TRUE) -> ()  [unwired: 2 in, 2 out]
            n103 = property on="Value" class="Slide (strict)"("Value"=w187, "Scale.Minimum"=w189, "Scale.Maximum"=w188, "Scale.Increment"=w186) -> ()  [unwired: 2 in, 2 out]
            n104 = property on="On/Off" class="Bool (strict)"("Visible"=w191) -> ()  [unwired: 2 in, 2 out]
            n105 = property on="Test Slider" class="Slide (strict)"("Visible"=w191) -> ()  [unwired: 2 in, 2 out]
            n106 = property on="Test Ring" class="Ring (strict)"("Visible"=w191) -> ()  [unwired: 2 in, 2 out]
            n107 = property on="Rev/Fwd" class="Clust (strict)"("Visible"=w191) -> ()  [unwired: 2 in, 2 out]
          }
          frame "Servo" {
            w203 = FALSE ("Visible")
            n108 = call <vilib>:"NT Read Number.vi"("Name"=w205) -> ("Numeric"=w204:dbl)  [unwired: 9 in, 1 out]
            n109 = property on="Test Slider" class="Slide (strict)"("Visible"=TRUE, "Scale.Maximum"=170.0 ("Scale.Range:Maximum")) -> ()  [unwired: 2 in, 2 out]
            n110 = local write "Test Slider"(w204) -> ()
            n111 = property on="Motor" class="Clust (strict)"("Visible"=w203) -> ()  [unwired: 2 in, 2 out]
            n112 = property on="Rev/Fwd" class="Clust (strict)"("Visible"=w203) -> ()  [unwired: 2 in, 2 out]
            n113 = property on="On/Off" class="Bool (strict)"("Visible"=w203) -> ()  [unwired: 2 in, 2 out]
            n114 = property on="Test Ring" class="Ring (strict)"("Visible"=w203) -> ()  [unwired: 2 in, 2 out]
          }
          frame "Relay", "Solenoid" {
            w206 = FALSE ("Visible")
            n115 = property on="Motor" class="Clust (strict)"("Visible"=w206) -> ()  [unwired: 2 in, 2 out]
            n116 = property on="Test Slider" class="Slide (strict)"("Visible"=w206) -> ()  [unwired: 2 in, 2 out]
            n117 = Search and Replace String(input string=w207, search string="/Value  **", replace string="/Direction") -> (result string=w213:string)  [unwired: 5 in, 3 out]
            n118 = property on="Test Ring" class="Ring (strict)"("Visible"=w206) -> ()  [unwired: 2 in, 2 out]
            n119 = call <vilib>:"NT Read String.vi"("Name"=w213) -> ("String"=w211:string)  [unwired: 9 in, 1 out]
            n120 = Equal?(x="Both directions", y=w211) -> (x = y?=w209:bool)
            n121 = Not(x=w209) -> (.not. x?=w210:bool)
            n122 = property on="Rev/Fwd" class="Clust (strict)"("Visible"=w209) -> ()  [unwired: 2 in, 2 out]
            n123 = property on="On/Off" class="Bool (strict)"("Visible"=w210, "Caption.Text"=w208) -> ()  [unwired: 2 in, 2 out]
          }
          frame "Compressor", "Digital Out" {
            w216 = FALSE ("Visible")
            # "Get direction and finish"
            n124 = property on="Motor" class="Clust (strict)"("Visible"=w216) -> ()  [unwired: 2 in, 2 out]
            n125 = property on="Test Slider" class="Slide (strict)"("Visible"=w216) -> ()  [unwired: 2 in, 2 out]
            n126 = property on="Test Ring" class="Ring (strict)"("Visible"=w216) -> ()  [unwired: 2 in, 2 out]
            n127 = property on="On/Off" class="Bool (strict)"("Visible"=TRUE, "Caption.Text"=w217) -> ()  [unwired: 2 in, 2 out]
            n128 = property on="Rev/Fwd" class="Clust (strict)"("Visible"=FALSE) -> ()  [unwired: 2 in, 2 out]
          }
          frame "Camera" {
            n129 = call <vilib>:"Get Last Path Segment.vi"("String in"=w224) -> ("String out"=w225:string)  [unwired: 10 in]
            n130 = property on="On/Off" class="Bool (strict)"("Visible"=FALSE) -> ()  [unwired: 2 in, 2 out]
            n131 = property on="Motor" class="Clust (strict)"("Visible"=FALSE) -> ()  [unwired: 2 in, 2 out]
            n132 = property on="Rev/Fwd" class="Clust (strict)"("Visible"=FALSE) -> ()  [unwired: 2 in, 2 out]
            n133 = case shown="\"White Balance  **\"" w225 {
              tunnel: w224 -> [w231 w240 w249 w258 w267 _ w273]
              tunnel: w223 -> [w229 w237 w246 w255 w264 _ _]
              frame "Size  **" {
                n134 = Index Array(array=w229) -> (element=w228:cluster{string[]})  [unwired: 1 in]
                n135 = call <vilib>:"NT Read String.vi"("Name"=w231) -> ("String"=w230:string)  [unwired: 9 in, 1 out]
                n136 = Unbundle(w228) -> (w226:string[])
                n137 = Match First String(2:w226, 3:w230) -> (0:w227:i32)  [unwired: 1 out]
                n138 = property on="Test Ring" class="Ring (strict)"("Value"=w227, "Strings []"=w226) -> ()  [unwired: 2 in, 2 out]
                n139 = property on="Test Ring" class="Ring (strict)"("Visible"=TRUE) -> ()  [unwired: 2 in, 2 out]
                n140 = property on="Test Slider" class="Slide (strict)"("Visible"=FALSE) -> ()  [unwired: 2 in, 2 out]
              }
              frame "White Balance  **" {
                n141 = Index Array(array=w237, index=1) -> (element=w238:cluster{string[]})
                n142 = call <vilib>:"NT Read String.vi"("Name"=w240) -> ("String"=w239:string)  [unwired: 9 in, 1 out]
                n143 = Unbundle(w238) -> (w235:string[])
                n144 = Match First String(2:w235, 3:w239) -> (0:w234:i32)  [unwired: 1 out]
                n145 = property on="Test Ring" class="Ring (strict)"("Value"=w234, "Strings []"=w235) -> ()  [unwired: 2 in, 2 out]
                n146 = property on="Test Ring" class="Ring (strict)"("Visible"=TRUE) -> ()  [unwired: 2 in, 2 out]
                n147 = property on="Test Slider" class="Slide (strict)"("Visible"=FALSE) -> ()  [unwired: 2 in, 2 out]
              }
              frame "Exposure  **" {
                n148 = Index Array(array=w246, index=2) -> (element=w247:cluster{string[]})
                n149 = call <vilib>:"NT Read String.vi"("Name"=w249) -> ("String"=w248:string)  [unwired: 9 in, 1 out]
                n150 = Unbundle(w247) -> (w243:string[])
                n151 = Match First String(2:w243, 3:w248) -> (0:w244:i32)  [unwired: 1 out]
                n152 = property on="Test Ring" class="Ring (strict)"("Value"=w244, "Strings []"=w243) -> ()  [unwired: 2 in, 2 out]
                n153 = property on="Test Ring" class="Ring (strict)"("Visible"=TRUE) -> ()  [unwired: 2 in, 2 out]
                n154 = property on="Test Slider" class="Slide (strict)"("Visible"=FALSE) -> ()  [unwired: 2 in, 2 out]
              }
              frame "Exposure Priority  **" {
                n155 = Index Array(array=w255, index=3) -> (element=w256:cluster{string[]})
                n156 = call <vilib>:"NT Read String.vi"("Name"=w258) -> ("String"=w257:string)  [unwired: 9 in, 1 out]
                n157 = Unbundle(w256) -> (w252:string[])
                n158 = Match First String(2:w252, 3:w257) -> (0:w253:i32)  [unwired: 1 out]
                n159 = property on="Test Ring" class="Ring (strict)"("Value"=w253, "Strings []"=w252) -> ()  [unwired: 2 in, 2 out]
                n160 = property on="Test Ring" class="Ring (strict)"("Visible"=TRUE) -> ()  [unwired: 2 in, 2 out]
                n161 = property on="Test Slider" class="Slide (strict)"("Visible"=FALSE) -> ()  [unwired: 2 in, 2 out]
              }
              frame "Color Enable  **" {
                n162 = Index Array(array=w264, index=4) -> (element=w265:cluster{string[]})
                n163 = call <vilib>:"NT Read String.vi"("Name"=w267) -> ("String"=w266:string)  [unwired: 9 in, 1 out]
                n164 = Unbundle(w265) -> (w261:string[])
                n165 = Match First String(2:w261, 3:w266) -> (0:w262:i32)  [unwired: 1 out]
                n166 = property on="Test Ring" class="Ring (strict)"("Value"=w262, "Strings []"=w261) -> ()  [unwired: 2 in, 2 out]
                n167 = property on="Test Ring" class="Ring (strict)"("Visible"=TRUE) -> ()  [unwired: 2 in, 2 out]
                n168 = property on="Test Slider" class="Slide (strict)"("Visible"=FALSE) -> ()  [unwired: 2 in, 2 out]
              }
              frame Default {
                n169 = property on="Test Ring" class="Ring (strict)"("Visible"=FALSE) -> ()  [unwired: 2 in, 2 out]
                n170 = property on="Test Slider" class="Slide (strict)"("Visible"=FALSE) -> ()  [unwired: 2 in, 2 out]
              }
              frame "Brightness  **", "Color Level  **", "Compression  **", "FPS  **", "Sharpness  **" {
                n171 = call <vilib>:"NT Read Number.vi"("Name"=w273) -> ("Numeric"=w272:dbl)  [unwired: 9 in, 1 out]
                n172 = local write "Test Slider"(w272) -> ()
                n173 = property on="Test Slider" class="Slide (strict)"("Visible"=TRUE, "Scale.Maximum"=100.0 ("Scale.Range:Maximum")) -> ()  [unwired: 2 in, 2 out]
                n174 = property on="Test Ring" class="Ring (strict)"("Visible"=FALSE) -> ()  [unwired: 2 in, 2 out]
              }
            }
          }
        }
        n175 = property on="Progress" class="Clust (strict)"("Visible"=FALSE) -> ()  [unwired: 2 in, 2 out]
      }
      event "Test Name": Mouse Enter {
        # "Populate the ring with the list of tests"
        n176 = event-data() -> ()  [unwired: 1 in, 1 out]
        n177 = call <vilib>:"NT Read String Array.vi"("Name"="TestMode/TestList") -> ("String Array"=w281:string[])  [unwired: 9 in, 1 out]
        n178 = Build Array (concatenate)("Select the test to run...", w281) -> (w280:string[])
        n179 = property on="Test Name" class="Ring (strict)"("Strings []"=w280) -> ()  [unwired: 2 in, 2 out]
      }
      event "Test Name": Value Change {
        w283 = FALSE ("Visible")
        # "Tell the robot the test name to run"
        n180 = event-data() -> ("NewVal"=w287:u16)  [unwired: 1 in]
        n181 = property on="Test Name" class="Ring (strict)"() -> ("Strings []"=w288:string[])  [unwired: 2 in, 2 out]
        n182 = local write "Progress"(T7 {"Test Progress"=0, "Test Progress Text"=""} ("Progress")) -> ()
        n183 = Index Array(array=w288, index=w287) -> (element=w286:string)
        n184 = call <vilib>:"NT Write String.vi"("String"=w286, "Name"="TestMode/TestName") -> ()  [unwired: 9 in, 1 out]
        n185 = property on="Progress" class="Clust (strict)"("Visible"=TRUE) -> ()  [unwired: 2 in, 2 out]
        n186 = property on="Motor" class="Clust (strict)"("Visible"=w283) -> ()  [unwired: 2 in, 2 out]
        n187 = property on="Test Slider" class="Slide (strict)"("Visible"=w283) -> ()  [unwired: 2 in, 2 out]
        n188 = property on="On/Off" class="Bool (strict)"("Visible"=w283) -> ()  [unwired: 2 in, 2 out]
        n189 = property on="Rev/Fwd" class="Clust (strict)"("Visible"=w283) -> ()  [unwired: 2 in, 2 out]
        n190 = property on="Test Ring" class="Ring (strict)"("Visible"=w283) -> ()  [unwired: 2 in, 2 out]
      }
      event "Listbox": Double Click {
        # "Shift clears all"
        # "Update symbols on the listbox"
        n191 = event-data() -> ("PlatMods.Shift"=w291:bool, "Row"=w293:i32)  [unwired: 1 in]
        n192 = case shown="True" w291 {
          tunnel: w293 -> [w297 _]
          tunnel: 1 -> [w296 _]
          frame False {
            n193 = property on="Listbox" class="LstBox (strict)"() -> ("Item Symbols"=w295:i32[])  [unwired: 2 in, 2 out]
            n194 = Replace Array Subset(array=w295, new element=w296, index=w297) -> (w294:i32[])
            n195 = property on="Listbox" class="LstBox (strict)"("Item Symbols"=w294) -> ()  [unwired: 2 in, 2 out]
          }
          frame True {
            w298 = 0 ("Top Row")
            n196 = property on="Listbox" class="LstBox (strict)"() -> ("Number of Rows"=w300:u32)  [unwired: 2 in, 2 out]
            n197 = Initialize Array(0, w300) -> (w299:i32[])
            n198 = property on="Listbox" class="LstBox (strict)"("Top Row"=w298, "Value"=w298, "Item Symbols"=w299) -> ()  [unwired: 2 in, 2 out]
          }
        }
      }
      event "Listbox": Key Down {
        # "Update symbols on the listbox\nLeft and right keys check and uncheck"
        n199 = event-data() -> ("VKey"=w304:T20)  [unwired: 1 in]
        n200 = case shown="\"Left\", \"Right\"" w304 {
          selector: w304 -> [w309 _]
          tunnel: eventvkey."Left" ("VKey") -> [w307 _]
          frame "Left", "Right" {
            n201 = Equal?(x=w307, y=w309) -> (x = y?=w308:bool)
            n202 = Select(t=0, s=w308, f=1) -> (s? t:f=w310:i32)
            n203 = property on="Listbox" class="LstBox (strict)"() -> ("Item Symbols"=w313:i32[])  [unwired: 2 in, 2 out]
            n204 = Replace Array Subset(array=w313, new element=w310, index="Listbox") -> (w312:i32[])
            n205 = property on="Listbox" class="LstBox (strict)"("Item Symbols"=w312) -> ()  [unwired: 2 in, 2 out]
          }
          frame Default {
          }
        }
      }
      event "DB Camera Config": Value Change {
        # "Show or hide the cluster of controls, store in ini file"
        n206 = event-data() -> ("NewVal"=w317:bool)  [unwired: 1 in]
        n207 = case shown="False" w317 {
          tunnel: w316 -> [w326 _]
          tunnel: [w319 w337] -> w315
          tunnel: w314 -> [w318 w337]
          frame False {
            w333 = "Camera"
            w336 = FALSE ("Visible")
            n208 = local read "Camera Settings"() -> (w325:T2)
            n209 = Index Array(array=w326) -> (element=w329:cluster{string[]})  [unwired: 1 in]
            n210 = Unbundle(w325) -> ("Frame Rate"=w324:i32, "Compression"=w323:i32, "Size"=w327:u16)
            n211 = Unbundle(w329) -> (w328:string[])
            n212 = Index Array(array=w328, index=w327) -> (element=w322:string)
            n213 = call-poly <vilib>:"Write Key.vi"("section"=w333, "value"=w322, "key"="Size", "refnum"=w318) -> ("refnum out"=w335:T18)  [unwired: 2 in, 5 out]
            n214 = call-poly <vilib>:"Write Key.vi"("section"=w333, "value"=w324, "key"="FrameRate", "refnum"=w335) -> ("refnum out"=w334:T18)  [unwired: 1 in, 6 out]
            n215 = property on="Camera Settings" class="Clust (strict)"("Visible"=w336) -> ()  [unwired: 2 in, 2 out]
            n216 = local write "DB Camera Config"(w336) -> ()
            n217 = call-poly <vilib>:"Write Key.vi"("section"=w333, "value"=w323, "key"="Compression", "refnum"=w334) -> ("refnum out"=w320:T18)  [unwired: 1 in, 6 out]
            n218 = call <vilib>:"Close Config Data.vi"("refnum"=w320) -> ("file path"=w321:path)  [unwired: 2 in, 8 out]
            n219 = call <vilib>:"Open Config Data.vi"("configuration file path"=w321) -> ("refnum"=w319:T18)  [unwired: 8 in, 2 out]
          }
          frame True {
            n220 = property on="Camera Settings" class="Clust (strict)"("Visible"=TRUE) -> ()  [unwired: 2 in, 2 out]
          }
        }
      }
      event "Camera Settings": Value Change {
        # "Update summary string when any elements of DB camera change"
        n221 = event-data() -> ("NewVal"=w350:T2)  [unwired: 1 in]
        n222 = Index Array(array=w346) -> (element=w345:cluster{string[]})  [unwired: 1 in]
        n223 = Unbundle(w350) -> ("Frame Rate"=w341:i32, "Compression"=w340:i32, "Size"=w343:u16)
        n224 = Unbundle(w345) -> (w344:string[])
        n225 = Index Array(array=w344, index=w343) -> (element=w342:string)
        n226 = Format Into String(format string="%s   %dfps   %d%%", w342, w341, w340) -> (resulting string=w347:string)  [unwired: 2 in, 1 out]
        n227 = Build Array(w347) -> (w348:string[])
        n228 = property on="DB Camera Config" class="Bool (strict)"("Strings [4]"=w348) -> ()  [unwired: 2 in, 2 out]
      }
      event "Motor.Enable": Value Change {
        # "When the test mode otor enable helper is set, update that\ntree row item's value"
        n229 = event-data() -> ("NewVal"=w356:bool)  [unwired: 1 in]
        n230 = Unbundle("Motor") -> ("Value"=w355:dbl)  [unwired: 1 out]
        n231 = Select(t=w355, s=w356, f=0.0) -> (s? t:f=w353:dbl)
        n232 = call <vilib>:"NT Write Number.vi"("Numeric"=w353, "Name"=w352) -> ()  [unwired: 9 in, 1 out]
      }
      event "Test Slider": Value Change {
        # "When the test mode slider helper is set, update that\ntree row item's value"
        n233 = event-data() -> ("NewVal"=w359:dbl)  [unwired: 1 in]
        n234 = call <vilib>:"NT Write Number.vi"("Numeric"=w359, "Name"=w360) -> ()  [unwired: 9 in, 1 out]
      }
      event "On/Off": Value Change {
        # "When the test mode on/off helper value is set, update that\ntree row item's value"
        n235 = event-data() -> ("NewVal"=w364:bool)  [unwired: 1 in]
        n236 = Boolean To (0,1)(Boolean=w364) -> (0, 1=w363:i16)
        n237 = call <vilib>:"NT Write Number.vi"("Numeric"=w363, "Name"=w362) -> ()  [unwired: 9 in, 1 out]
      }
      event "Rev/Fwd": Value Change {
        # "When the test mode helper value for relays is set, update that\ntree row item's value"
        n238 = event-data() -> ("NewVal.Forward"=w372:bool, "NewVal.Reverse"=w371:bool)  [unwired: 1 in]
        n239 = Boolean To (0,1)(Boolean=w372) -> (0, 1=w368:i16)
        n240 = Boolean To (0,1)(Boolean=w371) -> (0, 1=w370:i16)
        n241 = Negate(x=w370) -> (-x=w369:i16)
        n242 = Add(x=w368, y=w369) -> (x+y=w367:i16)
        n243 = call <vilib>:"NT Write Number.vi"("Numeric"=w367, "Name"=w366) -> ()  [unwired: 9 in, 1 out]
      }
      event "Test Ring": Value Change {
        # "When a test mode helper value is selected from the ring,\nset the tree item's variable to the string value"
        n244 = event-data() -> ("NewVal"=w376:u16)  [unwired: 1 in]
        n245 = property on="Test Ring" class="Ring (strict)"() -> ("Strings []"=w377:string[])  [unwired: 2 in, 2 out]
        n246 = Index Array(array=w377, index=w376) -> (element=w375:string)
        n247 = call <vilib>:"NT Write String.vi"("String"=w375, "Name"=w374) -> ()  [unwired: 9 in, 1 out]
      }
      event "Rec Mode": Value Change {
        # "Update globals for recording mode and path to read log from.\nClear when logging and let NetworkTables set path for vision to\nuse."
        n248 = event-data() -> ("NewVal"=w387:enum32{"Stop", "Record", "Playback"})  [unwired: 1 in]
        n249 = global write "WPI_DashboardLogging Global.vi" "Logging Filename"(path "") -> ()
        n250 = case shown="\"Playback\"" w387 {
          tunnel: w386 -> [_ w389 w397]
          tunnel: [_ _ w396] -> w383
          tunnel: [_ _ w395] -> _
          tunnel: w381 -> [_ _ w393]
          tunnel: cluster{i32, i32} {-250, 170} -> [_ _ w392]
          tunnel: [_ _ T21 {"Image Size"=TRUE, "Image Type"=TRUE, "Pixel Value"=TRUE, "ROI Information"=TRUE, "Zoom Factor"=FALSE} ("Image Information Shown:All Elements")] -> w379
          tunnel: [_ _ TRUE ("Zoom Factor")] -> w378
          frame Default {
          }
          frame "Stop", "Record" {
            # "Place Window too"
            n251 = invoke class="VI" method="FP.Close"(reference=w389) -> (reference out=w388:refnum<vi>)  [unwired: 2 in, 2 out]
            n252 = invoke class="VI" method="Abort VI"(reference=w388) -> ()  [unwired: 2 in, 3 out]
          }
          frame "Playback" {
            n253 = call "Open Playback Panel.vi"("Offset"=w392, "DB VI Ref"=w393, "Playback in"=w397) -> ("Playback out"=w394:refnum<vi>)  [unwired: 8 in]
            n254 = register-events(w394) -> (reference out=w396:refnum<event-registration>, error out=w395:errorcluster)  [unwired: 2 in]
          }
        }
        n255 = global write "WPI_DashboardLogging Global.vi" "Recording"(w387) -> ()
        n256 = property on="Camera Image" class="ImageControl"("Image Information Shown"=w379, "Image Information Visible"=w378) -> ()  [unwired: 2 in, 2 out]
        n257 = call <vilib>:"WPI_DashboardNT Log FieldName Cache.vi"("Operation"=enum16{"Lookup/Add", "Index", "Clear"}."Clear") -> ()  [unwired: 8 in, 3 out]
      }
      event Panel Close {
        w398 = enum32{"Stop", "Record", "Playback"}."Stop" ("Rec Mode")
        # "Playback window has been closed, abort"
        n258 = event-data() -> ()  [unwired: 1 in, 4 out]
        n259 = local write "Rec Mode"(w398) -> ()
        n260 = global write "WPI_DashboardLogging Global.vi" "Recording"(w398) -> ()
      }
      event Panel Close {
        # "Abort playback window and ourself"
        n261 = event-data() -> ()  [unwired: 1 in, 4 out]
        n262 = invoke class="VI" method="FP.Close"(reference=w403) -> (reference out=w402:refnum<vi>)  [unwired: 2 in, 2 out]
        n263 = invoke class="VI" method="Abort VI"(reference=w402) -> (error out=w401:errorcluster)  [unwired: 2 in, 2 out]
        n264 = invoke class="VI" method="Abort VI"(error in=w401) -> ()  [unwired: 2 in, 3 out]
      }
      event "Vision": Value Change {
        # "Enable/Disable Compression slider.\nHW USB is hard-coded into the camera"
        n265 = event-data() -> ("NewVal"=w409:u16)  [unwired: 1 in]
        n266 = Equal?(x=w409, y=u32 2 ("milliseconds to wait")) -> (x = y?=w407:bool)
        n267 = Select(t=T22."Disabled and Grayed Out" ("Disabled"), s=w407, f=T22."Enabled" ("Disabled")) -> (s? t:f=w404:T22)
        n268 = property on="Compression" class="Slide (strict)"("DisabledEnum"=w404) -> ()  [unwired: 2 in, 2 out]
      }
    }
  }
  n269 = while {
    tunnel: w38 -> [w412]
    i -> [w415]
    stop <- FALSE stop-if-true
    n270 = Wait (ms)(milliseconds to wait=u32 100) -> ()  [unwired: 1 out]
    n271 = case shown="\"Playback\"" "Rec Mode" {
      tunnel: w415 -> [_ _ w430]
      tunnel: [u32 2829099 ("Base Color") u32 11141120 ("Target Color") w419] -> w411
      frame "Stop", Default {
        # "Reset the color, extra updates don't cost much"
      }
      frame "Record" {
      }
      frame "Playback" {
        # "Playback"
        n272 = Quotient & Remainder(x=w430, y=u32 50 ("milliseconds to wait")) -> (x-y*floor(x/y)=w426:u32)  [unwired: 1 out]
        n273 = Divide(x=w426, y=u32 50 ("milliseconds to wait")) -> (x/y=w423:dbl)
        n274 = Multiply(x=6.283185307179586, y=w423) -> (x*y=w428:dbl)
        n275 = Sine(x=w428) -> (sin(x)=w427:dbl)
        n276 = Absolute Value(x=w427) -> (abs(x)=w420:dbl)
        n277 = call "Interpolate RGB Color.vi"("Proportion"=w420, "Target Color"=u32 30976, "Base Color"=u32 2829099) -> ("Result Color"=w419:u32)  [unwired: 8 in]
      }
    }
    n278 = property class="Pane"(reference=w412, "PaneColor"=w411) -> ()  [unwired: 1 in, 2 out]
  }
  n279 = TCP Create Listener(10:u16 1741 ("timeout ms (25000)")) -> (3:w1:refnum<k5>)  [unwired: 4 in, 2 out]
  n280 = while {
    tunnel: w1 -> [w432]
    stop <- FALSE stop-if-true
    n281 = TCP Wait On Listener(11:w432) -> (4:w431:refnum<k5>)  [unwired: 3 in, 4 out]
    n282 = local write "TCP"(w431) -> ()
  }
  n283 = property on="On/Off" class="Bool (strict)"("Visible"=w6) -> ()  [unwired: 2 in, 2 out]
  n284 = property on="Motor" class="Clust (strict)"("Visible"=w6) -> ()  [unwired: 2 in, 2 out]
  n285 = property on="Progress" class="Clust (strict)"("Visible"=w6) -> ()  [unwired: 2 in, 2 out]
  n286 = property on="Test Ring" class="Ring (strict)"("Visible"=w6) -> ()  [unwired: 2 in, 2 out]
  n287 = property on="Rev/Fwd" class="Clust (strict)"("Visible"=w6) -> ()  [unwired: 2 in, 2 out]
  n288 = property on="Camera Settings" class="Clust (strict)"("Visible"=w6) -> ()  [unwired: 2 in, 2 out]
  n289 = local write "DB Camera Config"(w6) -> ()
  n290 = global write "WPI_DashboardLogging Global.vi" "Recording"(w32) -> ()
  n291 = local write "Rec Mode"(w32) -> ()
